vi "daqmx_task_empty_test.vi"() -> ()   [LabVIEW 2013]
panel:
  out "x = y? 3":bool
  out "x = y? 2":bool
  out "x = y?":bool
  in  "Shock intensity AO task":refnum<k21>
  in  "Switch DI task":refnum<k21>
  in  "Code_LED DO task":refnum<k21>
  in  "Sound AO task":refnum<k21>
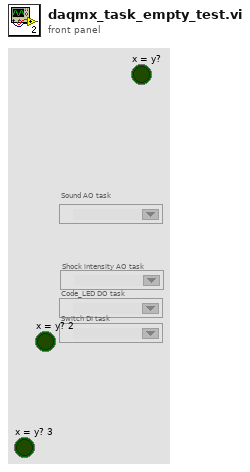
[diagram p1: front panel]
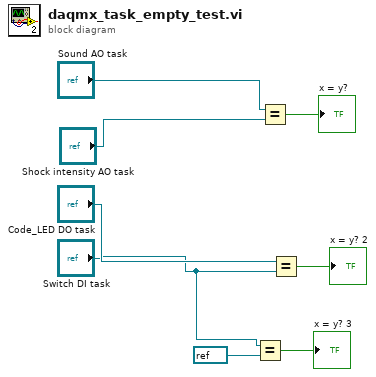
[diagram p0: block diagram]
diagram:
  n1 = Equal?(x="Switch DI task", y=refnum<k21> refnum) -> (x = y?=→"x = y? 3":bool)
  n2 = Equal?(x="Sound AO task", y="Shock intensity AO task") -> (x = y?=→"x = y?":bool)
  n3 = Equal?(x="Code_LED DO task", y="Switch DI task") -> (x = y?=→"x = y? 2":bool)
